vi "get ParentNode.vi"(8 "error in (no error)":errorcluster caption="错误输入（无错误）", 11 "PanelLinkNode输入":refnum<class "PanelLinkNode.lvclass">) -> (0 "error out":errorcluster caption="错误输出", 2 "ParentNode*":refnum<data-value>, 3 "PanelLinkNode输出":refnum<class "PanelLinkNode.lvclass">)   [LabVIEW 2013, in "PanelLinkNode.lvclass"]
uses:
  PanelLinkNode.lvclass
  PanelObject/PanelObject.lvclass
  PanelLinkNode.lvclass/PanelLinkNode.ctl
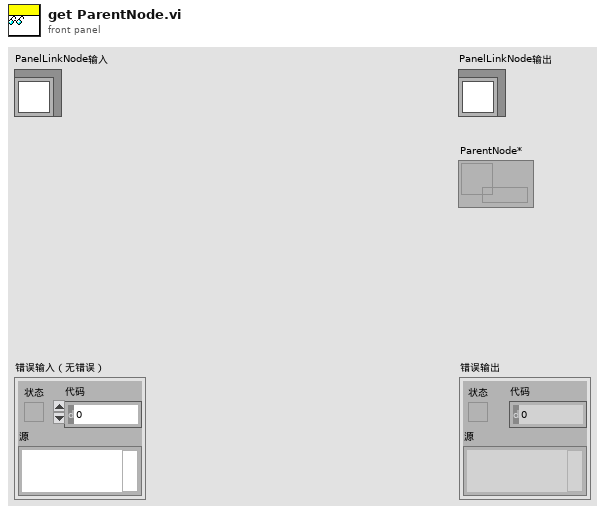
[diagram p1: front panel]
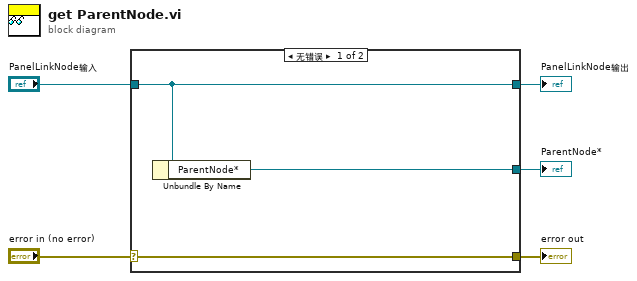
[diagram p0: block diagram]
diagram:
  n1 = case shown="无错误" "error in (no error)" {
    selector: "error in (no error)" -> [w8 w9]
    tunnel: [w8 w9] -> w4
    tunnel: [w7 w10] -> w2
    tunnel: "PanelLinkNode输入" -> [w7 w10]
    tunnel: [w6 _] -> w1
    frame No Error {
      n2 = Unbundle By Name(w7) -> ("ParentNode*"=w6:refnum<data-value>)
    }
    frame Error {
    }
  }
  "error out" <- w4
  "PanelLinkNode输出" <- w2
  "ParentNode*" <- w1
